vi "ReadFromTermoDat2.vi"(0 "Количество Термодатов":i32, 5 "Cluster":T6={"Baud Rate"=9600, "Parity"=0, "Flow Control"=0, "Timeout"=10000, "Mode"=enum."RTU", "VISA resource name"="", "Timeout 2"=5000, "Serial Parameters"={"Mode"=enum."RTU", "Slave Address"=0}, "Starting Address"=0, "Quantity"=1} {"Serial Parameters"."Slave Address" format="%.0x"; "Flow Control" items=["None", "XON/XOFF", "RTS/CTS", "XON/XOFF & RTS/CTS", "DTR/DSR", "XON/XOFF & DTR/DSR"]; "Parity" items=["None", "Odd", "Even", "Mark", "Space"]}) -> (10 "error out":errorcluster, 15 "output array":dbl[](array[numeric]))   [LabVIEW 2018]
uses:
  LW/Termodat_16K5/Control 2.ctl
  LW/Termodat_16K5/Control 4.ctl
  LW/Termodat_16K5/Control 3.ctl
  LW/Termodat_16K5/Control 1.ctl
  LW/Termodat_16K5/Control 5.ctl
panel:
  out "Exception Code":u8 format="%.0x"
  # "Параметры инициализации"
  # "Параметры чтения"
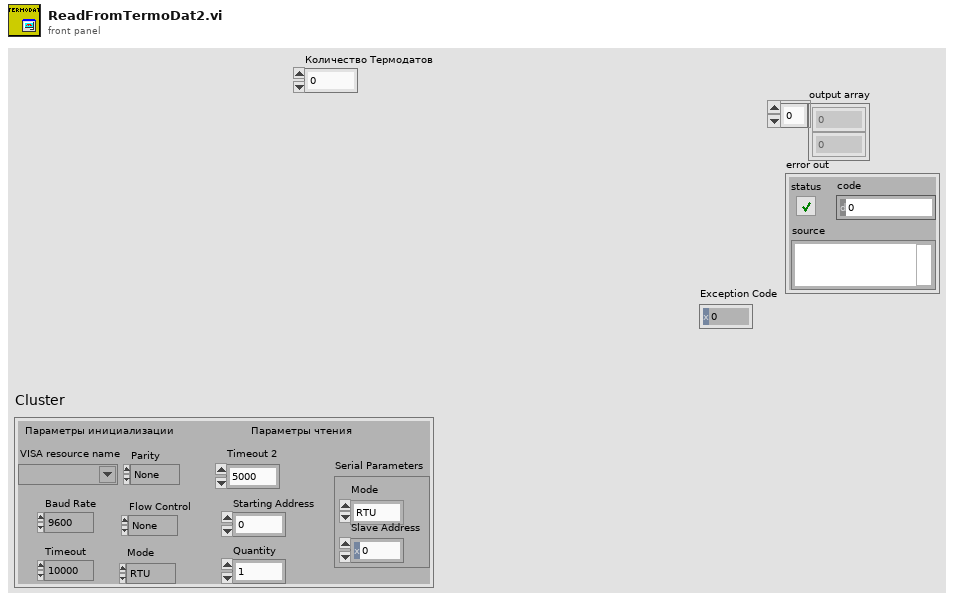
[diagram p1: front panel]
types:
  T1 = typedef "Control 2.ctl" = u32
  T2 = typedef "Control 4.ctl" = u32
  T3 = typedef "Control 3.ctl" = enum16{"RTU", "ASCII"}
  T4 = typedef "Control 1.ctl" = refnum<visa-resource-name>
  T5 = typedef "Control 5.ctl" = u32
  T6 = cluster{"Baud Rate":T1, "Parity":u16, "Flow Control":u16, "Timeout":T2, "Mode":T3, "VISA resource name":T4, "Timeout 2":T5, "Serial Parameters":cluster{"Mode":enum16{"RTU", "ASCII"}, "Slave Address":u8}, "Starting Address":u16, "Quantity":u16}
  T7 = cluster{"Mode":enum16{"RTU", "ASCII"}, "Slave Address":u8}
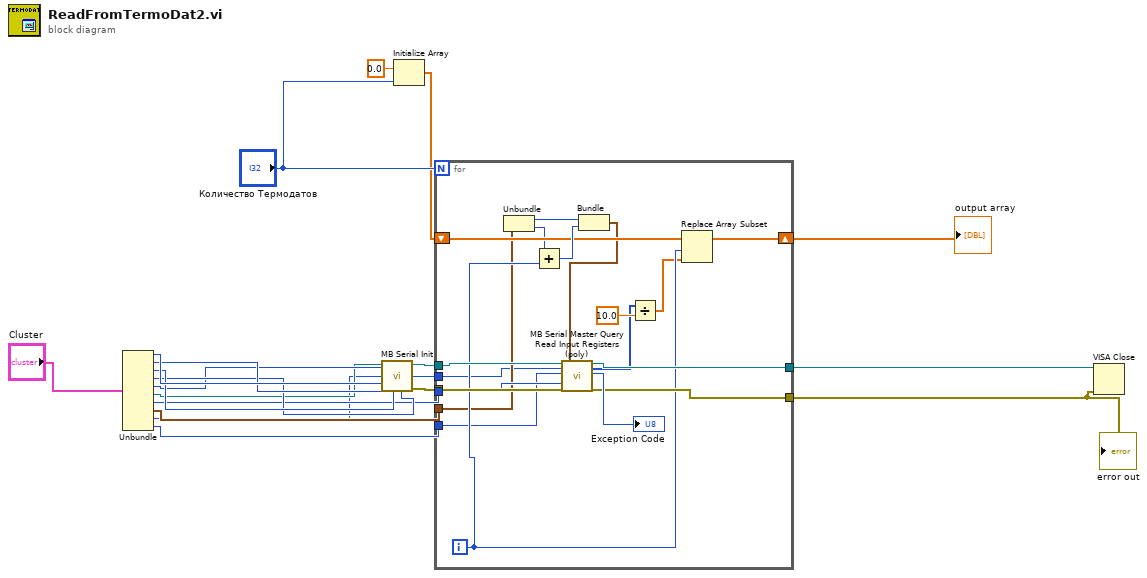
[diagram p0: block diagram]
diagram:
  n1 = Unbundle("Cluster") -> ("Baud Rate"=w10:T1, "Parity"=w9:u16, "Flow Control"=w8:u16, "Timeout"=w7:T2, "Mode"=w6:T3, "VISA resource name"=w5:T4, "Timeout 2"=w4:T5, "Serial Parameters"=w3:T7, "Starting Address"=w2:u16, "Quantity"=w1:u16)
  n2 = call <instrlib>:"MB Serial Init.vi"("Timeout"=w7, "Flow Control"=w8, "Mode"=w6, "Parity"=w9, "Baud Rate"=w10, "VISA resource name"=w5) -> ("error out"=w18:errorcluster, "VISA resource name out"=w19:refnum<visa-resource-name>)  [unwired: 4 in]
  n3 = Initialize Array(0.0 ("element"), "Количество Термодатов") -> (w13:dbl[])
  n4 = for {
    N: "Количество Термодатов" -> [_]
    tunnel: w19 -> [w37]
    tunnel: w18 -> [w38]
    tunnel: [w35] -> w17
    tunnel: [w34] -> w16
    shift-right: [w26] -> w12
    shift-left: w13 -> [w27]
    tunnel: w4 -> [w25]
    tunnel: w3 -> [w24]
    tunnel: w2 -> [w22]
    tunnel: w1 -> [w21]
    i -> [w31]
    n5 = Unbundle(w24) -> ("Mode"=w33:enum16{"RTU", "ASCII"}, "Slave Address"=w20:u8)
    n6 = Add(x=w20, y=w31) -> (x+y=w32:i32)
    n7 = Bundle("Mode"=w33, w32) -> (w23:cluster{"Mode":enum16{"RTU", "ASCII"}, i32})  [unwired: 1 in]
    n8 = call <instrlib>:"MB Serial Master Query Read Input Registers (poly).vi"("VISA resource name"=w37, "Starting Address"=w22, "Quantity"=w21, "Timeout"=w25, "error in"=w38, "Serial Parameters"=w23) -> ("VISA resource name out"=w34:refnum<visa-resource-name>, "Input Registers"=w29:u16[], "Exception Code"=→"Exception Code":u8, "error out"=w35:errorcluster)  [unwired: 10 in]
    n9 = Divide(x=w29, y=10.0) -> (x/y=w28:dbl[])
    n10 = Replace Array Subset(array=w27, new element=w28, index=w31) -> (w26:dbl[])
  }
  "output array" <- w12
  "error out" <- w17
  n11 = VISA Close(VISA resource name=w16, error in (no error)=w17) -> ()  [unwired: 1 out]
